vi "ExTestDevOutput.vi"() -> ()   [LabVIEW 2010]
panel:
  in  "stop":bool
  out "error out":errorcluster
  in  "error in (no error)":errorcluster
  # "ExTestDevOutput:\nThis example outputs in a loop to the TTL line\nthe out put should be a repeating ramp until the\nstop button is hit. The address is set for the \nPrinceton Instruments systems and TTL lines (0).\nNote: not all camera systems support TTL"
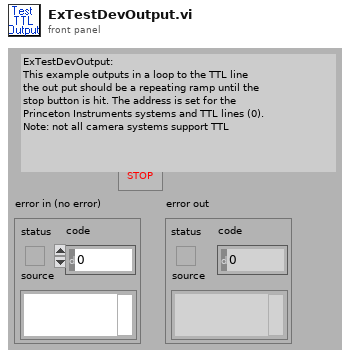
[diagram p1: front panel]
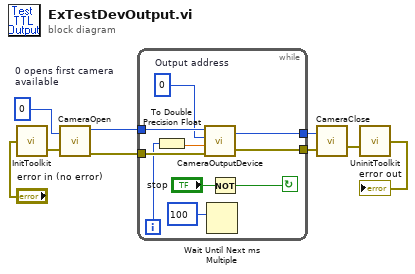
[diagram p0: block diagram]
diagram:
  w7 = 0  # 0 opens first camera  available
  n1 = call <userlib>:"InitToolkit.vi"("error in"="error in (no error)") -> ("error out"=w9:errorcluster)
  n2 = call <userlib>:"CameraOpen.vi"("error in"=w9, "Camera Device ID"=w7) -> ("error out"=w4:errorcluster, "Camera Handle"=w3:u32)
  n3 = while {
    tunnel: w4 -> [w19]
    tunnel: w3 -> [w18]
    tunnel: [w17] -> w2
    tunnel: [w16] -> w1
    i -> [w14]
    stop <- w11 continue-if-true
    w12 = 0  # Output address
    n4 = To Double Precision Float(number=w14) -> (double precision float=w13:dbl)
    n5 = call <userlib>:"CameraOutputDevice.vi"("error in"=w19, "Output value"=w13, "Output Address"=w12, "Camera Handle"=w18) -> ("error out"=w16:errorcluster, "Camera Handle"=w17:u32)
    n6 = Wait Until Next ms Multiple(millisecond multiple=100) -> ()  [unwired: 1 out]
    n7 = Not(x="stop") -> (.not. x?=w11:bool)
  }
  n8 = call <userlib>:"CameraClose.vi"("error in"=w1, "Camera Handle"=w2) -> ("error out"=w8:errorcluster)
  n9 = call <userlib>:"UninitToolkit.vi"("error in"=w8) -> ("error out"=→"error out":errorcluster)
